vi "CThread Get Execution State.vi"   [LabVIEW 2012, in "CThread.lvlib"]
uses:
  CThread.lvlib
  Core/CThread Thread Properties.ctl
  CRef/Interface/CRef Boolean.llb/Boolean CReference.ctl
  CRef/CRef.lvlib
  XNodes/terminalnode/CThread VI Terminal Node.xnode
  CRef/Interface/CRef Numeric.llb/I32 CReference.ctl
  Base/CThread Base - Get Execution State.vi
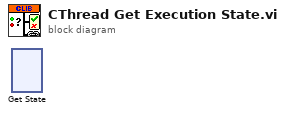
[diagram p0: block diagram]
diagram:
  n1 = xnode "Get State"() -> ()  [unwired: 1 in, 4 out]
